vi "Jiter Benchmark (RT).vi"() -> ()   [LabVIEW 2013]
doc: "This example uses an assembly-level call to obtain precise timestamps from RT targets. The purpose of this example is to gather timing information on a user's VI by running it for several iterations. The example obtains several consecutive 64-bit timestamps, which are stored in an array and used later to produce a histogram of execution time. This VI can self-calibrate by subtracting out the overhead of calling NI Get Timestamp.vi from the array of timing data.\n\nINSTRUCTIONS:\n1. Select a number of iterations and warmup iterations to exclude from the benchmark.\n2. Use calibration if you want to exclude the overhead of the timestamping operation.\n3. Go to the diagram and insert the code you want to benchmark."
uses:
  <vilib>/NI_Real-Time Target Support.lvlib
panel:
  in  "Tab Control":enum32{"Results", "Configure"}(tab)
  in  "Target Period":u32=2 caption="msec"
  out "Max jitter":dbl caption="usec" format="%.2f"
  out "Average period":dbl caption="usec" format="%.2f"
  in  "Calibrate?":bool
  in  "Warmup iterations":i32=10
  in  "Iterations":i32=500
  in  "stop":bool
  out "Execution Times":dbl[](graph)
  # "LabVIEW Real-Time Jitter Benchmark"
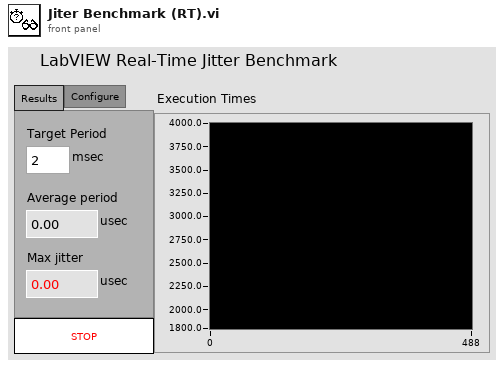
[diagram p1: front panel]
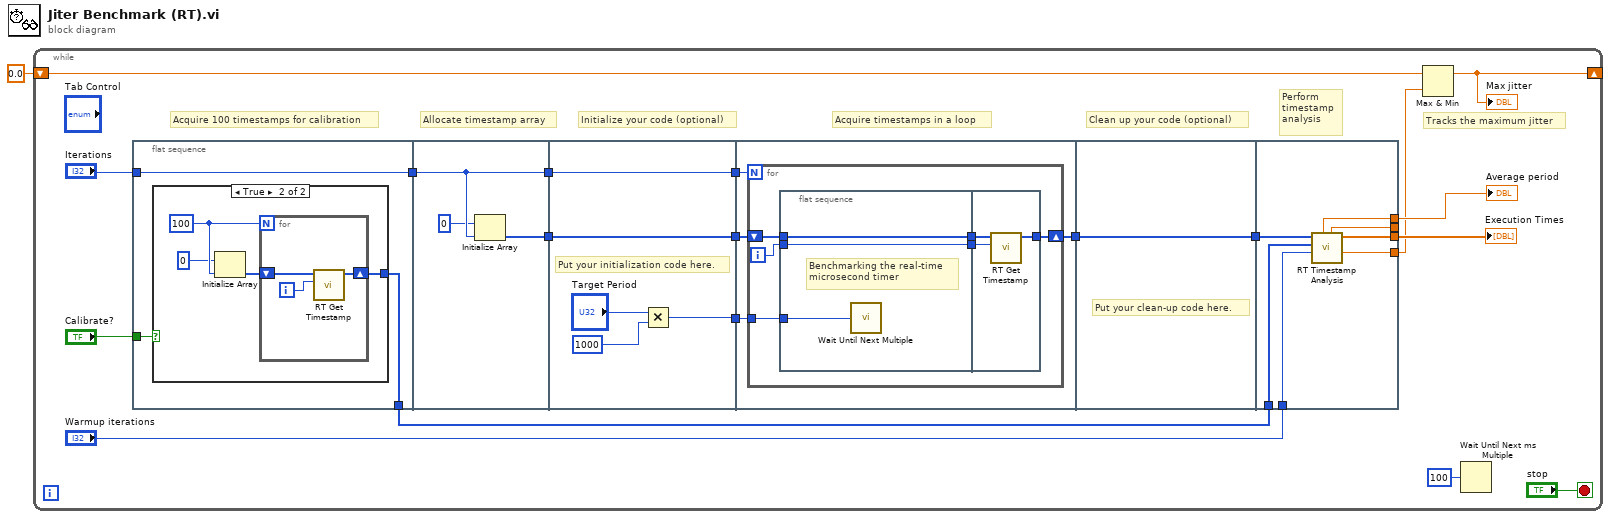
[diagram p0: block diagram]
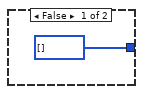
[diagram p2: hidden frame]
diagram:
  n1 = while {
    shift-right: [w4] -> _
    shift-left: 0.0 -> [w2]
    stop <- "stop" stop-if-true
    # "Tracks the maximum jitter"
    # "Perform timestamp analysis"
    # "Acquire timestamps in a loop"
    # "Clean up your code (optional)"
    # "Initialize your code (optional)"
    # "Allocate timestamp array"
    # "Acquire 100 timestamps for calibration"
    n2 = flat-sequence {
      tunnel: "Iterations" -> [w23]
      tunnel: [w23] -> w20
      tunnel: "Calibrate?" -> [w22]
      tunnel: [w21] -> w12
      tunnel: [w33] -> w19
      tunnel: [w34] -> w18
      tunnel: w20 -> [w33]
      tunnel: [w39] -> w17
      tunnel: [w38] -> w16
      tunnel: w19 -> [w39]
      tunnel: w18 -> [w38]
      tunnel: [w35] -> w15
      tunnel: [w43] -> w14
      tunnel: w17 -> [w42]
      tunnel: w16 -> [w41]
      tunnel: w15 -> [w40]
      tunnel: w14 -> [w56]
      tunnel: [w56] -> w13
      tunnel: w13 -> [w63]
      tunnel: w12 -> [w62]
      tunnel: [w61] -> w3
      tunnel: [w60] -> _
      tunnel: [w59] -> w10
      tunnel: "Warmup iterations" -> [w58]
      tunnel: [w57] -> w11
      frame #0 {
        n3 = case shown="True" w22 {
          tunnel: [u64[] [] w28] -> w21
          frame False {
          }
          frame True {
            w26 = 100
            n4 = Initialize Array(u64 0, w26) -> (w27:u64[])
            n5 = for {
              N: w26 -> [_]
              shift-right: [w29] -> w28
              shift-left: w27 -> [w30]
              i -> [w31]
              n6 = call <vilib>:"RT Get Timestamp.vi"("iteration"=w31, "timestamp array in"=w30) -> ("timestamp array out"=w29:u64[])  [unwired: 1 in, 8 out]
            }
          }
        }
      }
      frame #1 {
        n7 = Initialize Array(u64 0, w33) -> (w34:u64[])
      }
      frame #2 {
        # "Put your initialization code here."
        n8 = Multiply(x="Target Period", y=u32 1000 ("x")) -> (x*y=w35:u32)
      }
      frame #3 {
        n9 = for {
          N: w42 -> [_]
          shift-right: [w49] -> w43
          shift-left: w41 -> [w48]
          tunnel: w40 -> [w44]
          i -> [w47]
          n10 = flat-sequence {
            tunnel: w48 -> [w52]
            tunnel: [w52] -> w46
            tunnel: w47 -> [w51]
            tunnel: [w51] -> w45
            tunnel: w44 -> [w50]
            tunnel: [w55] -> w49
            tunnel: w46 -> [w53]
            tunnel: w45 -> [w54]
            frame #0 {
              # "Benchmarking the real-time\nmicrosecond timer"
              n11 = call "Wait Until Next Multiple"("Count(uSec)"=w50) -> ()  [unwired: 1 out]
            }
            frame #1 {
              n12 = call <vilib>:"RT Get Timestamp.vi"("iteration"=w54, "timestamp array in"=w53) -> ("timestamp array out"=w55:u64[])  [unwired: 1 in, 8 out]
            }
          }
        }
      }
      frame #4 {
        # "Put your clean-up code here."
      }
      frame #5 {
        n13 = call <vilib>:"RT Timestamp Analysis.vi"("warmup iterations"=w58, "calibration array"=w62, "timestamp array"=w63) -> ("max jitter (uS)"=w61:dbl, "execution times (uS)"=w59:dbl[], "standard deviation (uS)"=w60:dbl, "mean time (uS)"=w57:dbl)  [unwired: 1 in, 4 out]
      }
    }
    n14 = Max & Min(x=w2, y=w3) -> (max(x,y)=w4:dbl)  [unwired: 1 out]
    "Max jitter" <- w4
    n15 = Wait Until Next ms Multiple(millisecond multiple=u32 100) -> ()  [unwired: 1 out]
    "Execution Times" <- w10
    "Average period" <- w11
  }
